vi "Binary string to number.vi"(11 "Binaty string":string) -> (3 "Numeric":u32)   [LabVIEW 2019]
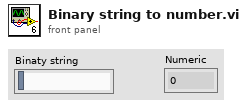
[diagram p1: front panel]
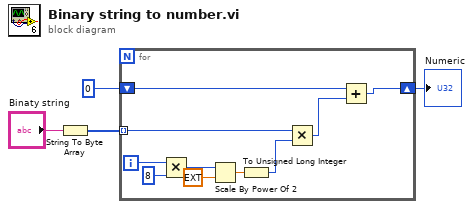
[diagram p0: block diagram]
diagram:
  n1 = String To Byte Array(string="Binaty string") -> (unsigned byte array=w4:u8[])
  n2 = for {
    tunnel: w4 -> [w10] mode=indexing
    shift-right: [w6] -> w2
    shift-left: u32 0 -> [w7]
    i -> [w13]
    n3 = Multiply(x=w13, y=8) -> (x*y=w14:i32)
    n4 = Scale By Power Of 2(n=w14, x=ext 1.0) -> (x*2^n=w9:ext)
    n5 = To Unsigned Long Integer(number=w9) -> (unsigned 32bit integer=w8:u32)
    n6 = Multiply(x=w10, y=w8) -> (x*y=w5:u32)
    n7 = Add(x=w7, y=w5) -> (x+y=w6:u32)
  }
  "Numeric" <- w2
